vi "Position (Reframed) Get.vi"(8 "error in (no error)":errorcluster, 10 "Frame Properties":T1) -> (0 "error out":errorcluster, 2 "Position (Reframed)":cluster{"x (m)":dbl, "y (m)":dbl, "z (mm)":dbl} {"z (mm)" format="%.1f"; "y (m)" format="%.1p"; "x (m)" format="%.1p"})   [LabVIEW 2019, in "Haptic Prog Interface.lvlib"]
doc: "Returns the horizontal xy-position of the haptic pen in nm, and the vertical z-position in mm. The horizontal position depends on the frame origin and frame size.\n\n<b>Position:</b> Returns a cluster of the x (nm), y (nm), and z (mm) positions of the pen."
uses:
  Haptic Prog Interface.lvlib
  dll_path.vi
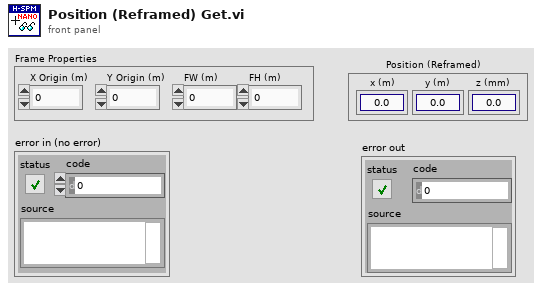
[diagram p1: front panel]
types:
  T1 = cluster{"X Origin (m)":dbl, "Y Origin (m)":dbl, "FW (m)":dbl, "FH (m)":dbl}
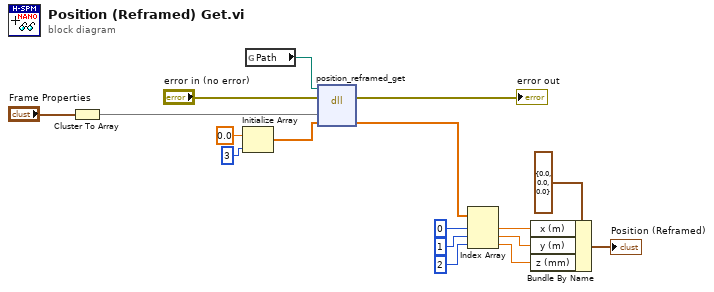
[diagram p0: block diagram]
diagram:
  n1 = Cluster To Array(cluster="Frame Properties") -> (array=w2:dbl[])
  n2 = Initialize Array(0.0 ("element"), 3 ("dimension size")) -> (w5:dbl[])
  n3 = global read "dll_path.vi" "Path"() -> (w17:path)
  n4 = dll-call lib="C:/Users/freem/Documents/GitHub/HapticSPM/Haptic-Programming-Interface/x64/Release/Haptic Programming Interface.dll" fn="position_reframed_get"(path in=w17, error in="error in (no error)", "frame_properties"=w2, "output"=w5) -> (error out=→"error out":errorcluster, "output"=w1:dbl[])  [unwired: 3 in, 1 out]
  n5 = Index Array(array=w1, index #1=0 ("index"), index #2=1 ("index"), index #3=2 ("index")) -> (element #1=w10:dbl, element #2=w9:dbl, element #3=w11:dbl)
  n6 = Bundle By Name(cluster=cluster{"x (m)":dbl, "y (m)":dbl, "z (mm)":dbl} {"x (m)"=0.0, "y (m)"=0.0, "z (mm)"=0.0} ("Position (Reframed)"), "x (m)"=w10, "y (m)"=w9, "z (mm)"=w11) -> (→"Position (Reframed)":cluster{"x (m)":dbl, "y (m)":dbl, "z (mm)":dbl})
